vi "FTW-CodeGen-GetTerms4.vi"(0 "State In":T2, 5 "XRef":refnum<vi>) -> (4 "Terms":T1(array[cluster]))   [LabVIEW 2012, in "FTW-JSON-Serialize.xnode"]
uses:
  FTW-JSON-Serialize.xnode
  FTW-CodeGen-State.ctl
panel:
  # "Inputs"
  # "Outputs"
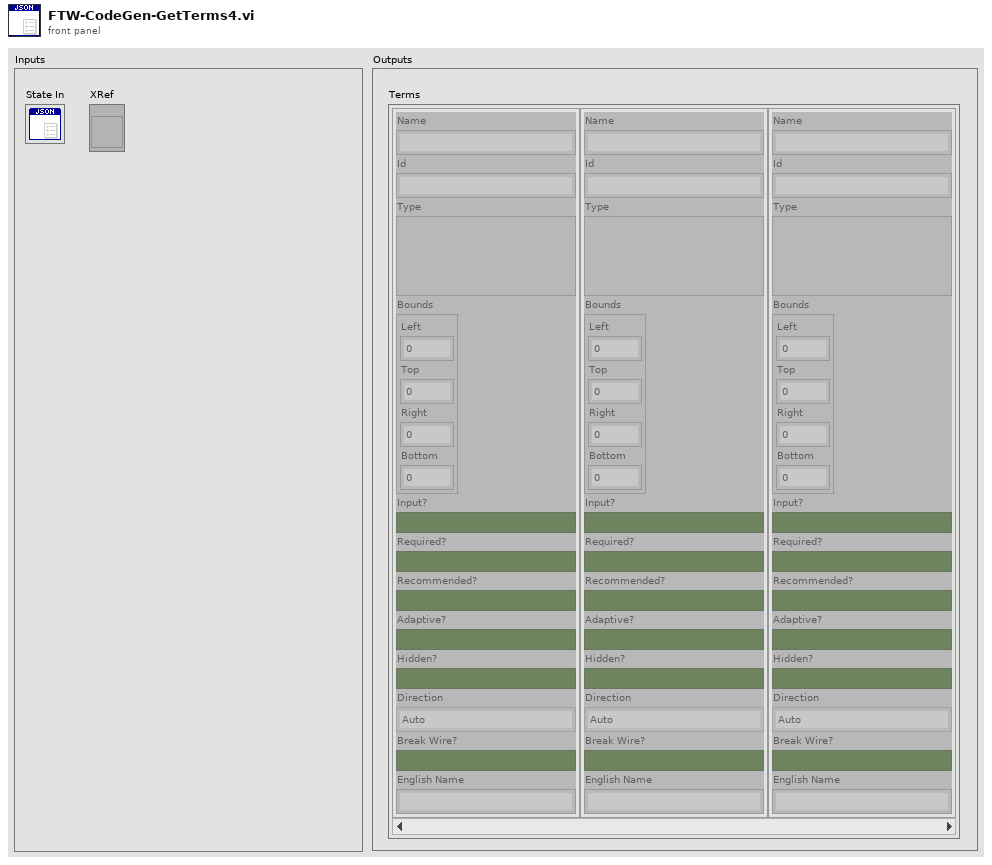
[diagram p1: front panel]
types:
  T1 = cluster{"Name":string, "Id":string, "Type":variant, "Bounds":cluster{"Left":i32, "Top":i32, "Right":i32, "Bottom":i32}, "Input?":bool, "Required?":bool, "Recommended?":bool, "Adaptive?":bool, "Hidden?":bool, "Direction":enum32{"Auto", "Up", "Down", "Left", "Right", "Center"}, "Break Wire?":bool, "English Name":string}[]
  T2 = typedef "FTW-JSON-Serialize.xnode/FTW-CodeGen-State.ctl" = cluster{"Prototype Filepath":path}
  T3 = cluster{"Name":string, "Id":string, "Type":variant, "Bounds":cluster{"Left":i32, "Top":i32, "Right":i32, "Bottom":i32}, "Input?":bool, "Required?":bool, "Recommended?":bool, "Adaptive?":bool, "Hidden?":bool, "Direction":enum32{"Auto", "Up", "Down", "Left", "Right", "Center"}, "Break Wire?":bool, "English Name":string}
  T4 = typedef "LVRectTypeDef.ctl" = cluster{"Left":i16, "Top":i16, "Right":i16, "Bottom":i16}
  T5 = enum16{"Invalid Wire Rule", "Required", "Recommended", "Optional", "Dynamic Dispatch"}[]
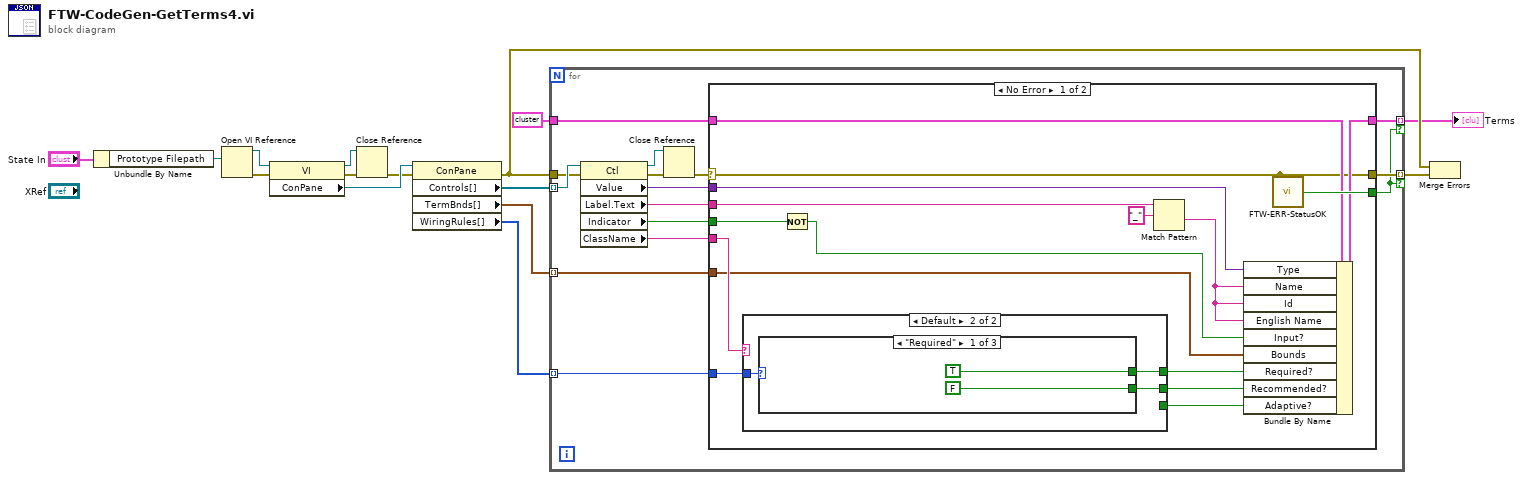
[diagram p0: block diagram]
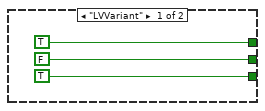
[diagram p2: hidden frame]
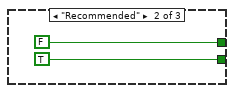
[diagram p3: hidden frame]
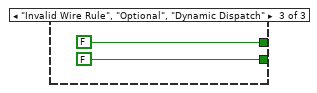
[diagram p4: hidden frame]
diagram:
  n1 = Unbundle By Name("State In") -> ("Prototype Filepath"=w4:path)
  n2 = Open VI Reference(vi path=w4) -> (vi reference=w2:refnum<vi>, error out=w3:errorcluster)  [unwired: 5 in]
  n3 = property class="VI"(reference=w2, error in=w3) -> (reference out=w8:refnum<vi>, error out=w10:errorcluster, "ConPane"=w15:refnum<vi>)
  n4 = Close Reference(reference=w8, error in (no error)=w10) -> (error out=w9:errorcluster)
  n5 = property class="ConPane"(reference=w15, error in=w9) -> (error out=w6:errorcluster, "Controls[]"=w14:refnum<vi>[], "TermBnds[]"=w11:T4[], "WiringRules[]"=w12:T5)  [unwired: 1 out]
  n6 = for {
    tunnel: w11 -> [w28] mode=indexing
    tunnel: w14 -> [w26] mode=indexing
    tunnel: w12 -> [w27] mode=indexing
    tunnel: T3 {"Name"="", "Id"="", "Type"=variant, "Bounds"={"Left"=0, "Top"=0, "Right"=0, "Bottom"=0}, "Input?"=FALSE, "Required?"=FALSE, "Recommended?"=FALSE, "Adaptive?"=FALSE, "Hidden?"=FALSE, "Direction"=enum."Auto", "Break Wire?"=FALSE, "English Name"=""} ("Term 4") -> [w30]
    tunnel: [w29] -> w5 mode=indexing if=w16
    tunnel: w6 -> [w21]
    tunnel: [w17] -> w7 mode=indexing if=w16
    n7 = property class="Ctl"(reference=w26, error in=w21) -> (reference out=w20:refnum<vi>, error out=w19:errorcluster, "Value"=w25:variant, "Label.Text"=w24:string, "Indicator"=w22:bool, "ClassName"=w23:string)
    n8 = Close Reference(reference=w20, error in (no error)=w19) -> (error out=w18:errorcluster)
    n9 = case shown="No Error" w18 {
      selector: w18 -> [w31 w59]
      tunnel: w30 -> [w45 w60]
      tunnel: [w44 w60] -> w29
      tunnel: w28 -> [w33 _]
      tunnel: w27 -> [w43 _]
      tunnel: w25 -> [w40 _]
      tunnel: w23 -> [w39 _]
      tunnel: w24 -> [w36 _]
      tunnel: w22 -> [w37 _]
      tunnel: [w46 _] -> w16
      tunnel: [w31 w59] -> w17
      frame No Error {
        n10 = case shown="Default" w39 {
          tunnel: w43 -> [_ w52]
          tunnel: [TRUE w51] -> w42
          tunnel: [FALSE w50] -> w41
          tunnel: [TRUE _] -> w38
          frame "LVVariant" {
          }
          frame Default {
            n11 = case shown="\"Required\"" w52 {
              tunnel: [TRUE FALSE FALSE] -> w51
              tunnel: [FALSE TRUE FALSE] -> w50
              frame "Required" {
              }
              frame "Recommended" {
              }
              frame "Invalid Wire Rule", "Optional", "Dynamic Dispatch" {
              }
            }
          }
        }
        n12 = Not(x=w37) -> (.not. x?=w32:bool)
        n13 = Match Pattern(string=w36, regular expression="_") -> (after substring=w34:string)  [unwired: 1 in, 3 out]
        n14 = Bundle By Name(cluster=w45, "Type"=w40, "Name"=w34, "Id"=w34, "English Name"=w34, "Input?"=w32, "Bounds"=w33, "Required?"=w42, "Recommended?"=w41, "Adaptive?"=w38) -> (w44:T3)
        n15 = call "FTW-ERR-StatusOK.vi"("error to check"=w31) -> ("Status OK?"=w46:bool)
      }
      frame Error {
      }
    }
  }
  "Terms" <- w5
  n16 = Merge Errors(w6, w7) -> ()  [unwired: 1 out]
